vi "PopAll.vi"(11 "POTTypedCircularBuffer in":refnum<class "POTTypedCircularBuffer.lvclass">) -> (2 "Flushed Buffer":T1[](array[typedef]), 3 "POTTypedCircularBuffer out":refnum<class "POTTypedCircularBuffer.lvclass">)   [LabVIEW 2024, in "POTTypedCircularBuffer.lvclass"]
uses:
  POTTypedCircularBuffer.lvclass
  Type.ctl
  POTTypedCircularBuffer.lvclass/POTTypedCircularBuffer.ctl
  ReadCount.vi
  Reorder.vi
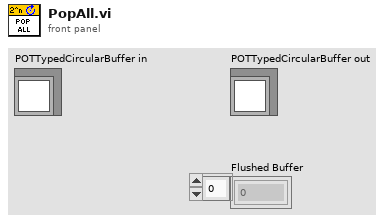
[diagram p1: front panel]
types:
  T1 = typedef "POTTypedCircularBuffer.lvclass/Type.ctl" = i32
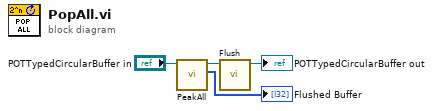
[diagram p0: block diagram]
diagram:
  n1 = call "PeakAll.vi"("POTTypedCircularBuffer in"="POTTypedCircularBuffer in") -> ("Copied Buffer"=→"Flushed Buffer":T1[], "POTTypedCircularBuffer out"=w4:refnum<class "POTTypedCircularBuffer.lvclass">)  [unwired: 9 in]
  n2 = call "Flush.vi"("POTTypedCircularBuffer in"=w4) -> ("POTTypedCircularBuffer out"=→"POTTypedCircularBuffer out":refnum<class "POTTypedCircularBuffer.lvclass">)  [unwired: 10 in]
